vi "Main Loop.vi"(8 "error in (no error)":errorcluster, 10 "Chart Notifier":refnum<notifier>, 11 "Message Queues":T1) -> (0 "error out":errorcluster)   [LabVIEW 2018, in "4-20mA Module.lvlib" / "4-20mA Module Engine.lvlib"]
uses:
  4-20mA Module Engine.lvlib
  Pressure Regulator/Controls/4-20mA Message Queues.ctl
  support/Message Queue/Message Cluster.ctl
  State Cluster.ctl
  State Enum.ctl
  Pressure Transmitter/Pressure Transmitter Device Settings.ctl
  Pressure Reg Module/Pressure Regulator Device Settings.ctl
  Measure Instrument/PID 1 Parameters Cluster.ctl
  Pressure Regulator/Controls/4-20mA Display Cluster.ctl
  <vilib>/Platform/TimedLoop/XDataNode/timing_clust.ctl
  <vilib>/Platform/TimedLoop/XDataNode/nitl_modes.ctl
  <vilib>/Platform/TimedLoop/XDataNode/wakeup.ctl
  Tag VIs/Tag FGV Operation Enum.ctl
  Pressure Regulator/Controls/4-20mA Module Settings Cluster.ctl
  support/Message Queue/Enqueue Message (Single).vi
  <vilib>/Utility/error.llb/Error Cluster From Error Code.vi
  <vilib>/Platform/TimedLoop/XDataNode/XDataNode.xnode
  <vilib>/ErrorRing/Error Ring.xnode
  support/Message Queue/Message Queue.lvlib
  <vilib>/Platform/TimedLoop/XDataNode/XDNodeRunTimeDep.lvlib
  Shared Variables/Dynamic Shared Variables.lvlib
  Pressure Transmitter/Pressure Transmitter Library.lvlib
  Pressure Reg Module/Pressure Regulator Library.lvlib
  Pressure Regulator/4-20mA Module.lvlib
panel:
  out "Period (s)":dbl format="%_4g"
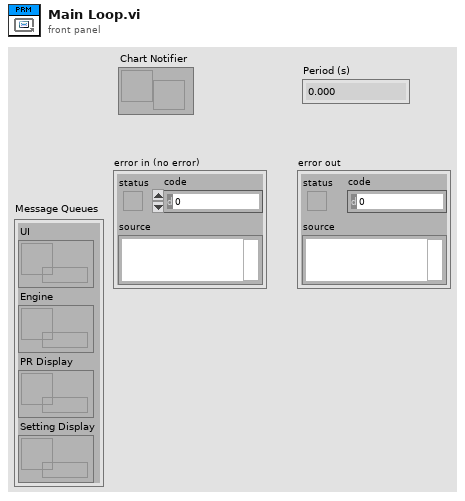
[diagram p1: front panel]
types:
  T1 = typedef "4-20mA Module.lvlib/4-20mA Message Queues.ctl" = cluster{"UI":refnum<queue>, "Engine":refnum<queue>, "PR Display":refnum<queue>, "Setting Display":refnum<queue>}
  T2 = typedef "4-20mA Module.lvlib/4-20mA Display Cluster.ctl" = cluster{"Input 4-20":dbl, "Output 4-20":dbl, "Cycle Period":dbl, "Status":enum16{"Off", "On", "Not Initialized"}}
  T3 = typedef "XDNodeRunTimeDep.lvlib/timing_clust.ctl" = cluster{"Expected End [f-1]":u64, "Actual End [f-1]":u64, "Finished Late? [f-1]":bool, "Expected End [i-1]":u64, "Actual End [i-1]":u64, "Finished Late? [i-1]":bool, "Expected Start [i]":u64, "Actual Start [i]":u64, "Expected Start [f]":u64, "Actual Start [f]":u64, "Source Name":string, "Structure Name":string, "Period":i64, "Deadline":i64, "Offset":i64, "Start":i64, "Priority":i32, "Timeout":i32, "Mode":T4, "Wakeup Reason":T5, "Error":errorcluster, "Source Type":string, "Secondary Source Type":string, "Global End Time":u64, "Global Start Time":u64, "Frame Duration":u64, "Iteration Duration":u64, "Assigned CPU":i32, "I/O Scan Engine Mode":u32}
  T4 = typedef "XDNodeRunTimeDep.lvlib/nitl_modes.ctl" = enum32{"No Change", "Process missed periods, maintain original phase", "Discard missed periods, maintain original phase", "Process missed periods, ignore original phase", "Discard missed periods, ignore original phase"}
  T5 = typedef "XDNodeRunTimeDep.lvlib/wakeup.ctl" = enum32{"Normal", "Aborted", "Asynchronous wakeup", "Timing source error", "Timed loop error", "Timeout"}
  T6 = cluster{"enable? (F)":bool, "name":string, "alarm on":bool, "priority":u32, "ack type":enum16{"Auto", "User", "None", "Each Occurrence"}, "area":string, "description":string, "log? (T)":bool}
  T7 = typedef "Tag FGV Operation Enum.ctl" = enum16{"Init", "Set Notification Queue", "Create Tag", "Commit", "Write Tag (Numeric)", "Write Tag (Boolean)", "Read All Tags", "Read One Tag", "Delete Tag Category", "Set Alarm Parameters (Numeric)", "Set Alarm Parameters (Boolean)", "Enable All Alarms", "Disable All Alarms", "Delete All Tags", "Read Alarms", "Ack Alarm"}
  T8 = enum32{"u32BitField", "bool", "double", "string", "int8", "uint8", "int16", "uint16", "int32", "uint32", "int64", "uint64", "single", "double waveform", "int16 waveform", "array of boolean", "array of int8", "array of uint8", "array of int16", "array of uint16", "array of int32", "array of uint32", "array of int64", "array of uint64", "array of single", "array of double", "array of double waveform", "array of int16 waveform", "array of string", "variant", "timestamp", "fixed point", "custom"}
  T9 = typedef "4-20mA Module.lvlib/4-20mA Module Engine.lvlib/State Enum.ctl" = enum16{"Measuring", "Idle", "Paused"}
  T10 = typedef "4-20mA Module.lvlib/4-20mA Module Settings Cluster.ctl" = cluster{"Cycle Period":dbl, "PID 2 Parameters":cluster{"Input Device":enum16{"Default", "4-20mA"}, "Output Device":enum16{"Default", "Equilibar Pressure Reg", "Flow Regulator"}, "Setpoint":dbl, "PID gains":cluster{"proportional gain (Kc)":dbl, "integral time (Ti, min)":dbl, "derivative time (Td, min)":dbl}, "output range":cluster{"output low":dbl, "output high":dbl}}, "Manual Entry":dbl, "Auto?":bool, "4-20mA Input Settings":T11, "4-20mA Out Settings":T12, "Input Channel Tag Name ":string}
  T11 = typedef "Pressure Transmitter Library.lvlib/Pressure Transmitter Device Settings.ctl" = cluster{"Input Channel ":u16}
  T12 = typedef "Pressure Regulator Library.lvlib/Pressure Regulator Device Settings.ctl" = cluster{"Output DAQ Task":refnum<k21>}
  T13 = typedef "4-20mA Module.lvlib/4-20mA Module Engine.lvlib/State Cluster.ctl" = cluster{"State":T9, "Start Time":timestamp, "Configuration":cluster{"Cycle Period":dbl, "PID 2 Parameters":cluster{"Input Device":enum16{"Default", "4-20mA"}, "Output Device":enum16{"Default", "Equilibar Pressure Reg", "Flow Regulator"}, "Setpoint":dbl, "PID gains":cluster{"proportional gain (Kc)":dbl, "integral time (Ti, min)":dbl, "derivative time (Td, min)":dbl}, "output range":cluster{"output low":dbl, "output high":dbl}}, "Manual Entry":dbl, "Auto?":bool, "4-20mA Input Settings":T11, "4-20mA Out Settings":T12, "Input Channel Tag Name ":string}, "Current Time":timestamp, "PID 1 Parameters":T14, "First Iteration":bool, "Data":cluster{"4-20mA Input":dbl, "PID 2 Process Variable":dbl, "PID 2 Output":dbl, "4-20mA Output":dbl}, "Process Name":string, "Pump On?":enum16{"Off", "On", "Not Initialized"}, "Input Error":bool, "Output Error":bool, "Log Started":bool, "Current Setpoint":dbl}
  T14 = typedef "PID 1 Parameters Cluster.ctl" = cluster{"Setpoint":dbl, "PID gains":cluster{"proportional gain (Kc)":dbl, "integral time (Ti, min)":dbl, "derivative time (Td, min)":dbl}}
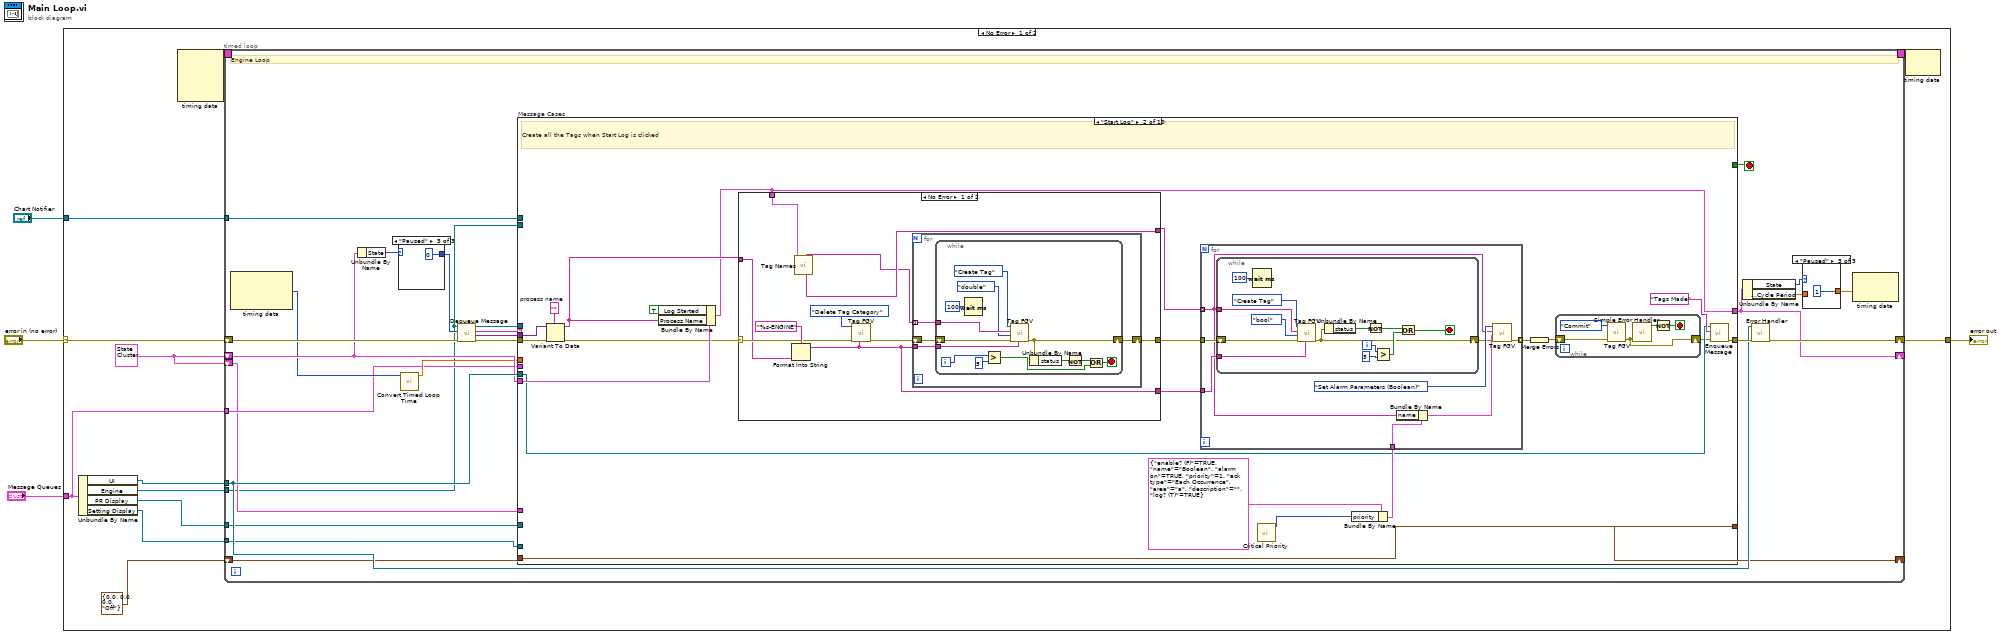
[diagram p0: block diagram]
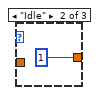
[diagram p3: hidden frame]
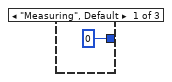
[diagram p4: hidden frame]
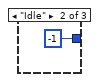
[diagram p5: hidden frame]
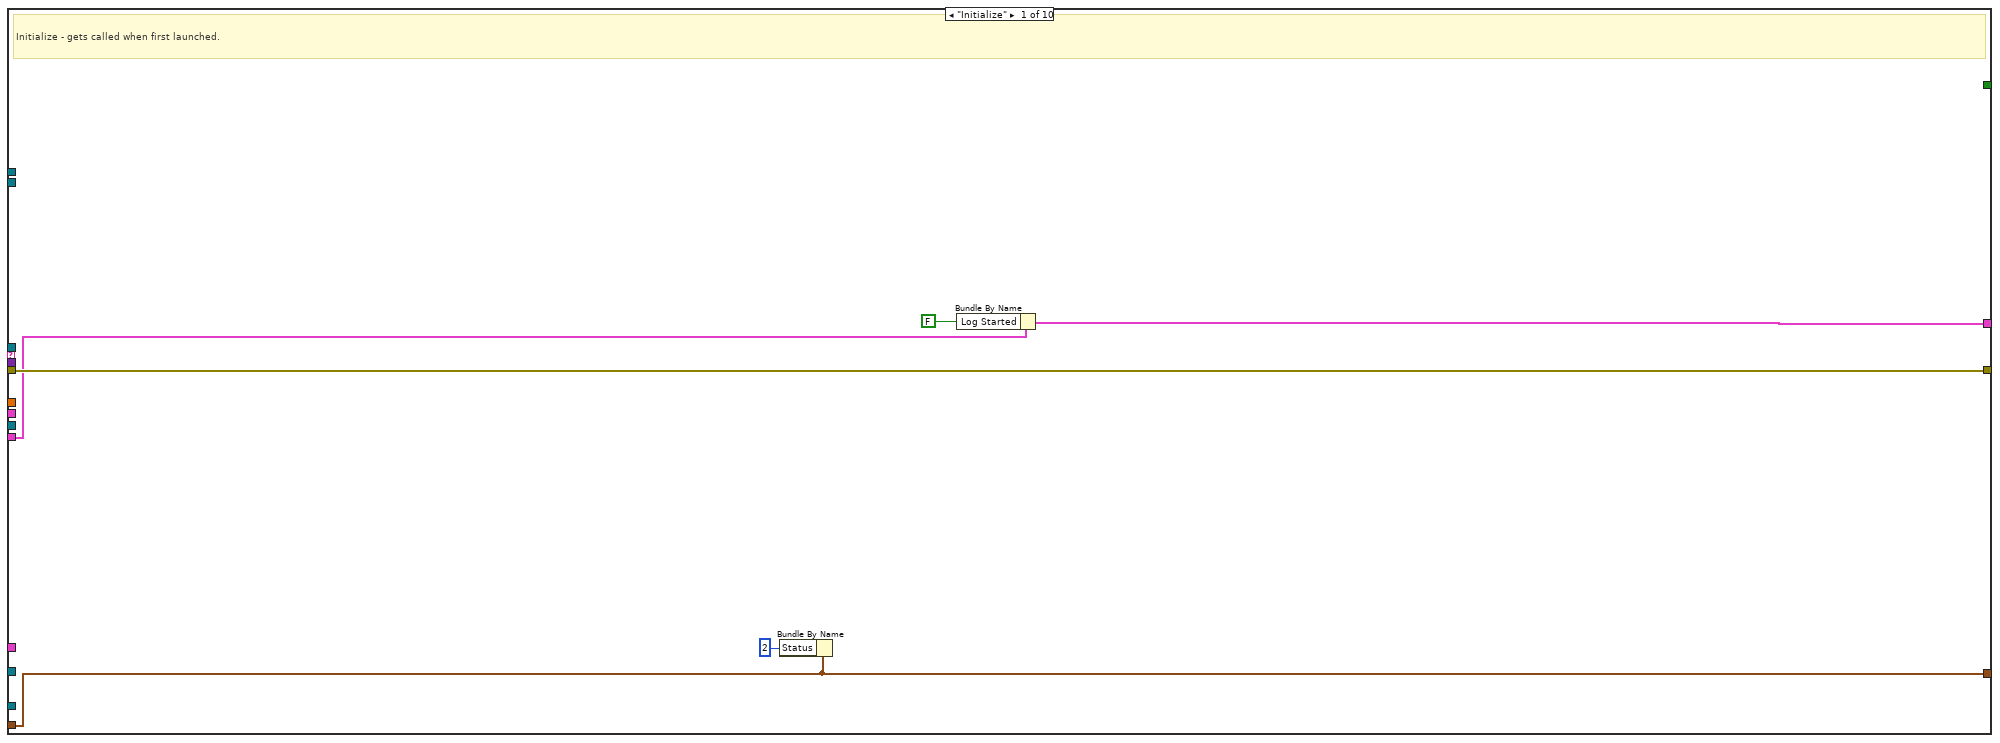
[diagram p6: hidden frame]
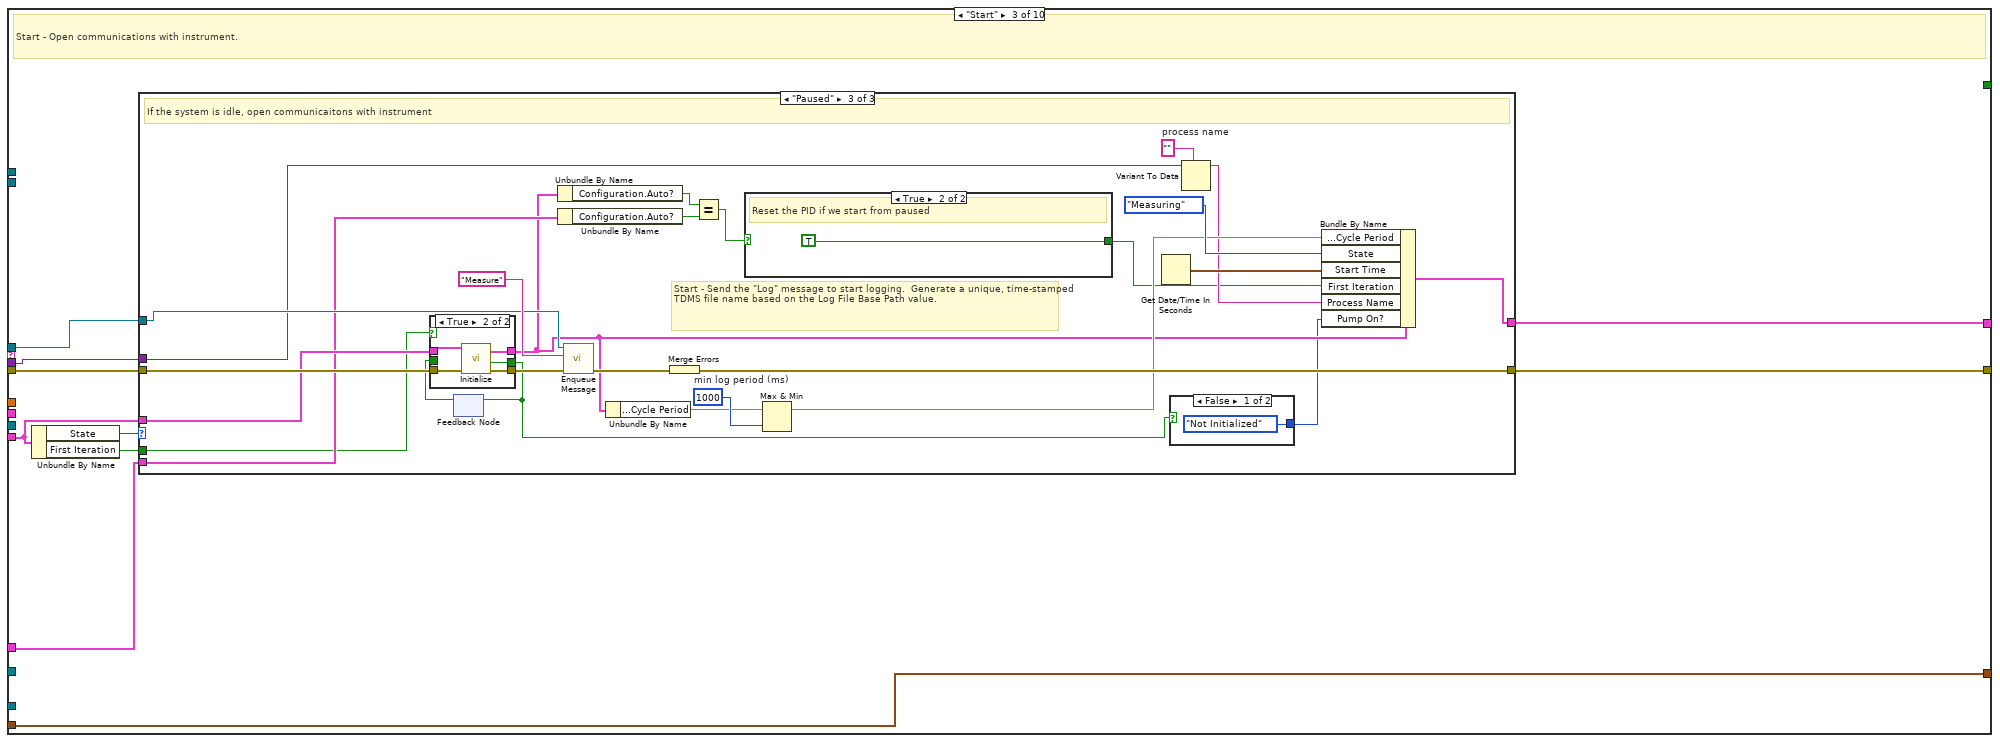
[diagram p8: hidden frame]
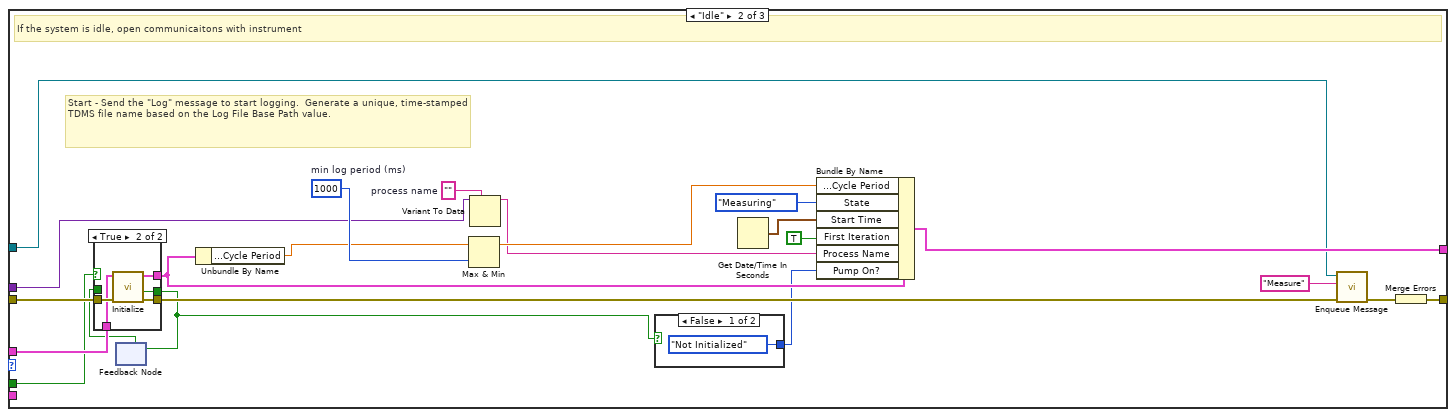
[diagram p10: hidden frame]
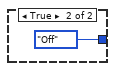
[diagram p12: hidden frame]
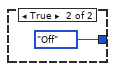
[diagram p14: hidden frame]
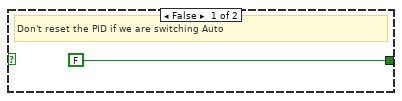
[diagram p15: hidden frame]
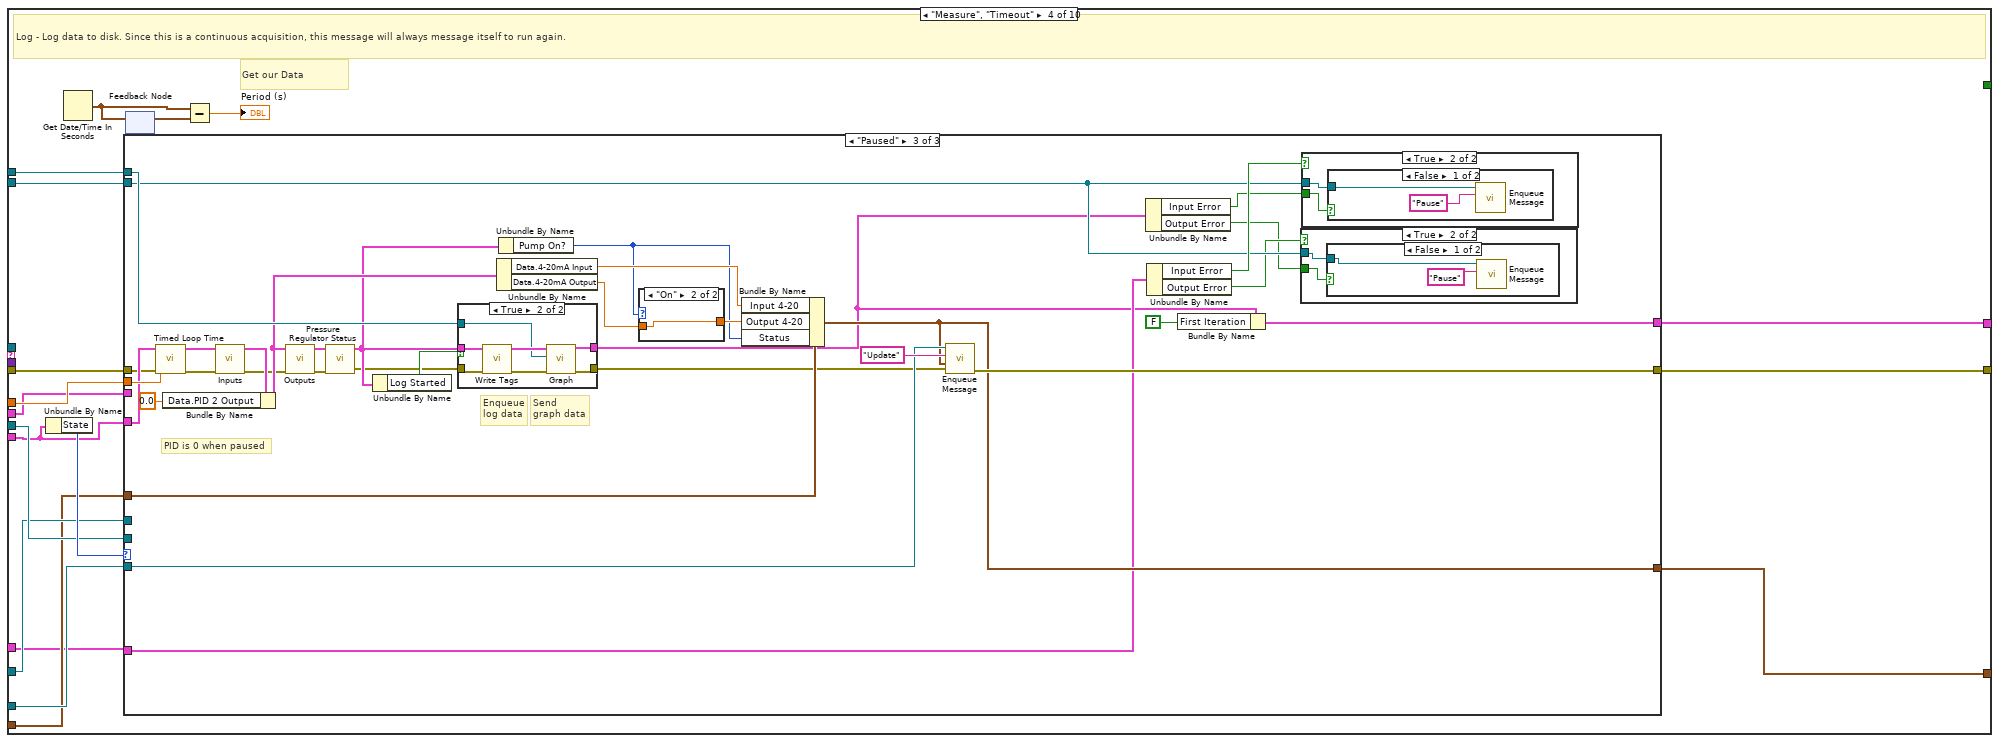
[diagram p16: hidden frame]
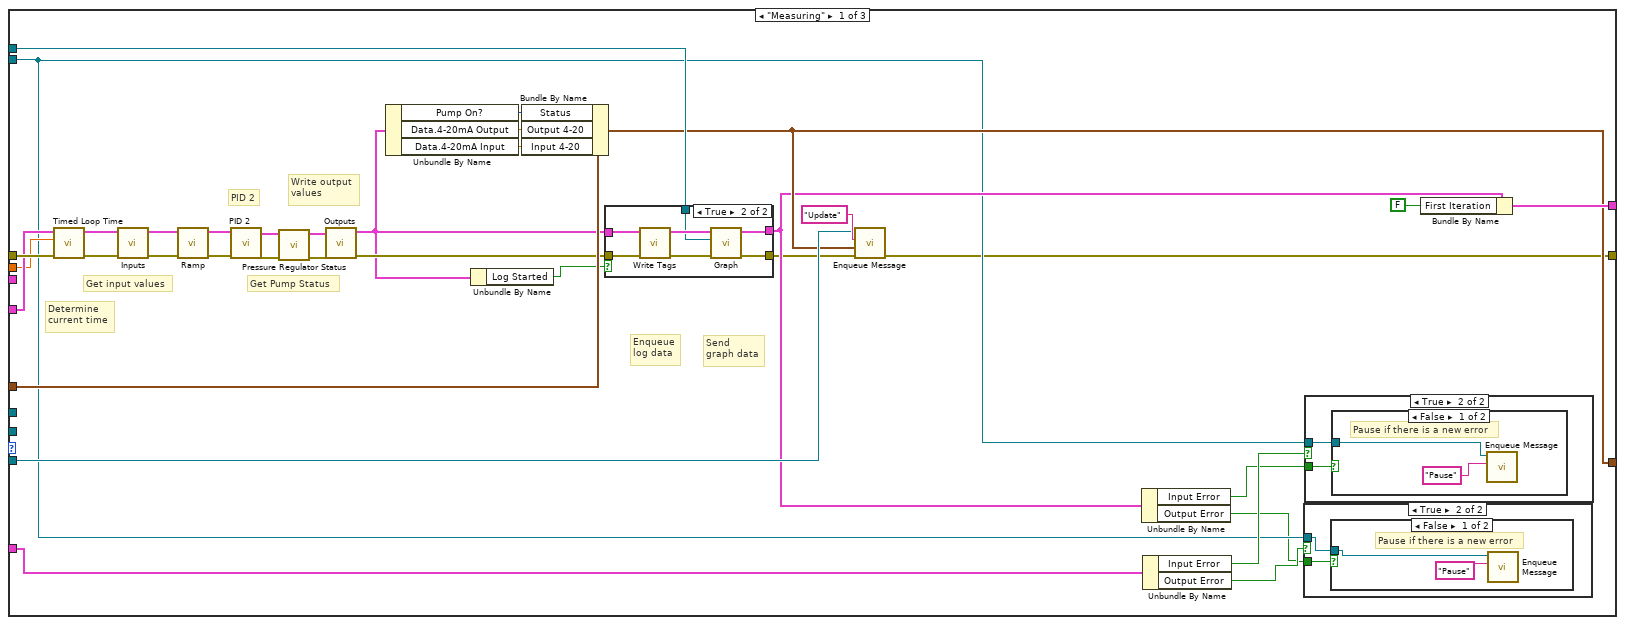
[diagram p17: hidden frame]
diagram:
  n1 = case shown="No Error" "error in (no error)" {
    selector: "error in (no error)" -> [w15 w454]
    tunnel: "Message Queues" -> [w11 _]
    tunnel: [w16 w454] -> w3
    tunnel: "Chart Notifier" -> [w9 _]
    frame No Error {
      w6 = T13 {"State"=enum."Idle", "Start Time"=timestamp(0 s since 1904-01-01), "Configuration"={"Cycle Period"=0.0, "PID 2 Parameters"={"Input Device"=enum."4-20mA", "Output Device"=enum."Equilibar Pressure Reg", "Setpoint"=0.0, "PID gains"={"proportional gain (Kc)"=1.0, "integral time (Ti, min)"=0.01, "derivative time (Td, min)"=0.0}, "output range"={"output low"=0.0, "output high"=100.0}}, "Manual Entry"=0.0, "Auto?"=TRUE, "4-20mA Input Settings"={"Input Channel "=0}, "4-20mA Out Settings"={"Output DAQ Task"=""}, "Input Channel Tag Name "=""}, "Current Time"=timestamp(0 s since 1904-01-01), "PID 1 Parameters"={"Setpoint"=0.0, "PID gains"={"proportional gain (Kc)"=1.0, "integral time (Ti, min)"=0.01, "derivative time (Td, min)"=0.0}}, "First Iteration"=FALSE, "Data"={"4-20mA Input"=0.0, "PID 2 Process Variable"=0.0, "PID 2 Output"=0.0, "4-20mA Output"=0.0}, "Process Name"="", "Pump On?"=enum."Off", "Input Error"=FALSE, "Output Error"=FALSE, "Log Started"=FALSE, "Current Setpoint"=0.0} ("State")
      n2 = Unbundle By Name(w11) -> ("UI"=w14:refnum<queue>, "Engine"=w10:refnum<queue>, "PR Display"=w8:refnum<queue>, "Setting Display"=w7:refnum<queue>)
      n3 = node-c288() -> (w13:T3)  [unwired: 4 in]
      n4 = timed-loop {
        tunnel: w10 -> [w19]
        shift-right: [w17] -> _
        shift-left: w6 -> [w34]
        shift-right: [w36] -> w16
        shift-left: w15 -> [w42]
        tunnel: w14 -> [w35]
        timing: w13 -> [_]
        timing-out: [_] -> w12
        tunnel: w11 -> [w26]
        tunnel: w9 -> [w25]
        tunnel: w8 -> [w24]
        tunnel: w7 -> [w23]
        shift-right: [w22] -> _
        shift-left: T2 {"Input 4-20"=0.0, "Output 4-20"=0.0, "Cycle Period"=0.0, "Status"=enum."Off"} ("PRM Display Cluster") -> [w18]
        shift-left: w6 -> [w21]
        stop <- w20 stop-if-true
        # "Engine Loop"
        n5 = node-c288() -> (w28:i64)  [unwired: 1 in, 2 out]
        n6 = Unbundle By Name(w34) -> ("State"=w33:T9)
        n7 = case shown="\"Paused\"" w33 {
          tunnel: [0 ("timeout in ms (-1)") -1 ("timeout in ms (-1)") 0 ("timeout in ms (-1)")] -> w32
          frame "Measuring", Default {
          }
          frame "Idle" {
          }
          frame "Paused" {
          }
        }
        n8 = call "Convert Timed Loop Time.vi"("Actual Start [i]"=w28) -> ("ET since start (s)"=w27:dbl)  [unwired: 10 in]
        n9 = call "Dequeue Message.vi"("error in (no error)"=w42, "timeout in ms (-1)"=w32, "Message Queue"=w19) -> ("error out"=w41:errorcluster, "Message Data"=w39:variant, "Message"=w40:string, "dup Message Queue"=w38:refnum<queue>)  [unwired: 5 in]
        n10 = case "Message Cases" shown="\"Start Log\"" w40 {
          selector: w40 -> [_ _ _ _ _ _ _ _ _ w443]
          tunnel: w38 -> [_ _ w143 _ w362 _ _ w430 _ _]
          tunnel: w41 -> [w59 w77 w142 w231 w351 w377 w424 w433 w440 _]
          tunnel: [w59 w63 w144 w232 w355 w381 w422 w435 w439 w444] -> w37
          tunnel: w34 -> [w58 w76 w139 w230 w350 w379 w421 w426 w437 w441]
          tunnel: [_ _ _ _ _ _ _ TRUE _ _] -> w20
          tunnel: w39 -> [_ w78 w140 _ _ _ w425 _ _ _]
          tunnel: w35 -> [_ w64 _ w233 w361 w386 _ w434 _ _]
          tunnel: w27 -> [_ _ _ w229 _ _ _ _ _ _]
          tunnel: w26 -> [_ _ _ w228 _ _ _ _ _ _]
          tunnel: w25 -> [_ _ _ w224 _ _ _ _ _ _]
          tunnel: w24 -> [_ _ _ w223 w353 _ _ _ _ _]
          tunnel: w23 -> [_ _ _ w222 w354 w383 _ _ _ _]
          tunnel: w18 -> [w55 w80 w138 w221 w352 w380 w423 w427 w438 w442]
          tunnel: [w55 w80 w138 w220 w352 w380 w423 w427 w438 w442] -> w22
          tunnel: w21 -> [_ _ w137 w219 _ _ _ _ _ _]
          tunnel: w19 -> [_ _ _ w218 _ _ _ _ _ _]
          tunnel: [w56 w62 w135 w217 w349 w374 w418 w426 w437 w441] -> w17
          frame "Initialize" {
            # "Initialize - gets called when first launched."
            n11 = Bundle By Name(cluster=w55, "Status"=u16 2) -> ()  [unwired: 1 out]
            n12 = Bundle By Name(cluster=w58, "Log Started"=FALSE) -> (w56:T13)
          }
          frame "Start Log" {
            w79 = ""  # process name
            # "Create all the Tags when Start Log is clicked"
            n13 = Variant To Data(error in=w77, type=w79, Variant=w78) -> (data=w74:string, error out=w75:errorcluster)
            n14 = Bundle By Name(cluster=w76, "Log Started"=TRUE, "Process Name"=w74) -> (w62:T13)
            n15 = case shown="No Error" w75 {
              selector: w75 -> [w113 w134]
              tunnel: [w116 w134] -> w69
              tunnel: w74 -> [w111 _]
              tunnel: [w110 _] -> w70
              tunnel: [w109 _] -> w67
              tunnel: w62 -> [w108 _]
              frame No Error {
                n16 = Format Into String(format string="%s-ENGINE", w111) -> (resulting string=w109:string)  [unwired: 2 in, 1 out]
                n17 = call "Tag Names.vi"("State in"=w108) -> ("All Boolean Tags"=w110:string[], "All  Numeric Tags"=w107:string[])  [unwired: 8 in, 1 out]
                n18 = call "Tag FGV.vi"("Tag Category"=w109, "error in (no error)"=w113, "Operation"=Tag_FGV_Operation_Enum."Delete Tag Category") -> ("error out"=w112:errorcluster)  [unwired: 3 in, 5 out]
                n19 = for {
                  tunnel: w107 -> [w120] mode=indexing
                  shift-right: [w118] -> w116
                  shift-left: w112 -> [w119]
                  tunnel: w109 -> [w117]
                  n20 = while {
                    tunnel: w120 -> [w132]
                    tunnel: w117 -> [w129]
                    shift-right: [w128] -> w118
                    shift-left: w119 -> [w130]
                    i -> [w123]
                    stop <- w121 stop-if-true
                    n21 = Wait (ms)(milliseconds to wait=u32 100) -> ()  [unwired: 1 out]
                    n22 = Greater?(x=w123, y=5 ("x")) -> (0:w122:bool)
                    n23 = call "Tag FGV.vi"("Tag Category"=w129, "error in (no error)"=w130, "Data"=T8."double" ("data type"), "Tag Name"=w132, "Operation"=Tag_FGV_Operation_Enum."Create Tag") -> ("error out"=w128:errorcluster)  [unwired: 1 in, 5 out]
                    n24 = Unbundle By Name(w128) -> ("status"=w127:bool)
                    n25 = Not(x=w127) -> (.not. x?=w125:bool)
                    n26 = Or(x=w125, y=w122) -> (x .or. y?=w121:bool)
                  }
                }
              }
              frame Error {
              }
            }
            n27 = call "Critical Priority.vi"() -> ("critical priority"=w72:i32)  [unwired: 11 in]
            n28 = Bundle By Name(cluster=T6 {"enable? (F)"=TRUE, "name"="Boolean", "alarm on"=TRUE, "priority"=1, "ack type"=enum."Each Occurrence", "area"="a", "description"="", "log? (T)"=TRUE} ("Boolean alarm settings"), "priority"=w72) -> (w71:T6)
            n29 = for {
              tunnel: w71 -> [w93]
              tunnel: [w92] -> w68 mode=indexing
              tunnel: w70 -> [w86] mode=indexing
              tunnel: w69 -> [w88]
              tunnel: w67 -> [w89]
              n30 = while {
                tunnel: w86 -> [w105]
                tunnel: w89 -> [w102]
                shift-right: [w94] -> w87
                shift-left: w88 -> [w103]
                i -> [w97]
                stop <- w95 stop-if-true
                n31 = Wait (ms)(milliseconds to wait=u32 100) -> ()  [unwired: 1 out]
                n32 = call "Tag FGV.vi"("Tag Category"=w102, "error in (no error)"=w103, "Data"=T8."bool" ("data type"), "Tag Name"=w105, "Operation"=Tag_FGV_Operation_Enum."Create Tag") -> ("error out"=w94:errorcluster)  [unwired: 1 in, 5 out]
                n33 = Unbundle By Name(w94) -> ("status"=w101:bool)
                n34 = Not(x=w101) -> (.not. x?=w99:bool)
                n35 = Greater?(x=w97, y=5 ("x")) -> (0:w96:bool)
                n36 = Or(x=w99, y=w96) -> (x .or. y?=w95:bool)
              }
              n37 = Bundle By Name(cluster=w93, "name"=w86) -> (w91:T6)
              n38 = call "Tag FGV.vi"("error in (no error)"=w87, "Data"=w91, "Tag Name"=w86, "Operation"=Tag_FGV_Operation_Enum."Set Alarm Parameters (Boolean)") -> ("error out"=w92:errorcluster)  [unwired: 2 in, 5 out]
            }
            n39 = Merge Errors(w68) -> (w61:errorcluster)
            n40 = while {
              shift-right: [w83] -> w60
              shift-left: w61 -> [w84]
              stop <- w81 stop-if-true
              n41 = call "Tag FGV.vi"("error in (no error)"=w84, "Operation"=Tag_FGV_Operation_Enum."Commit") -> ("error out"=w83:errorcluster)  [unwired: 4 in, 5 out]
              n42 = call <vilib>:"Simple Error Handler.vi"("error in (no error)"=w83) -> ("error?"=w82:bool)  [unwired: 4 in, 4 out]
              n43 = Not(x=w82) -> (.not. x?=w81:bool)
            }
            n44 = call-poly "Enqueue Message.vi"("error in (no error)"=w60, "Message"="Tags Made", "Message Queue"=w64) -> ("error out"=w63:errorcluster)  [unwired: 7 in, 1 out]
          }
          frame "Start" {
            # "Start - Open communications with instrument."
            n45 = Unbundle By Name(w139) -> ("State"=w141:T9, "First Iteration"=w136:bool)
            n46 = case shown="\"Paused\"" w141 {
              tunnel: [w145 w168 w204] -> w144
              tunnel: w143 -> [_ w159 w195]
              tunnel: w142 -> [w145 w157 w193]
              tunnel: w139 -> [w146 w156 w192]
              tunnel: [w146 w166 w202] -> w135
              tunnel: w140 -> [_ w154 w190]
              tunnel: w137 -> [_ _ w186]
              tunnel: w136 -> [_ w147 w181]
              frame "Measuring", Default {
                # "The system is already running. Ignore the \"Start\" message."
              }
              frame "Idle" {
                w155 = ""  # process name
                w163 = 1000  # min log period (ms)
                # "Start - Send the \"Log\" message to start logging.  Generate a unique, time-stamped TDMS file name based on the Log File Base Path value."
                # "If the system is idle, open communicaitons with instrument"
                n47 = feedback #1() -> (w149:bool)  [unwired: 1 in]
                n48 = case shown="True" w147 {
                  tunnel: w157 -> [w170 w176]
                  tunnel: w156 -> [w171 w175]
                  tunnel: [w171 w174] -> w152
                  tunnel: [w170 w173] -> w151
                  tunnel: [w169 w172] -> w148
                  tunnel: w149 -> [w169 _]
                  frame False {
                  }
                  frame True {
                    n49 = call "Initialize.vi"("error in (no error)"=w176, "State in"=w175) -> ("error out"=w173:errorcluster, "Pump Initialized"=w172:bool, "State out"=w174:T13)  [unwired: 7 in]
                  }
                }
                n50 = feedback-in #1(w148) -> ()
                n51 = Unbundle By Name(w152) -> ("Configuration.Cycle Period"=w162:dbl)
                n52 = Max & Min(x=w162, y=w163) -> (max(x,y)=w161:dbl)  [unwired: 1 out]
                n53 = Variant To Data(type=w155, Variant=w154) -> (data=w153:string)  [unwired: 1 in, 1 out]
                n54 = case shown="False" w148 {
                  tunnel: [enum16{"Off", "On", "Not Initialized"}."Not Initialized" ("Pump On?") enum16{"Off", "On", "Not Initialized"}."Off" ("Pump On?")] -> w150
                  frame False {
                  }
                  frame True {
                  }
                }
                n55 = Get Date/Time In Seconds() -> (seconds since 1Jan1904=w160:timestamp)
                n56 = Bundle By Name(cluster=w152, "Configuration.Cycle Period"=w161, "State"=State_Enum."Measuring", "Start Time"=w160, "First Iteration"=TRUE, "Process Name"=w153, "Pump On?"=w150) -> (w166:T13)
                n57 = call-poly "Enqueue Message.vi"("error in (no error)"=w151, "Message"="Measure", "Message Queue"=w159) -> ("error out"=w164:errorcluster)  [unwired: 7 in, 1 out]
                n58 = Merge Errors(w164) -> (w168:errorcluster)
              }
              frame "Paused" {
                w191 = ""  # process name
                w199 = 1000  # min log period (ms)
                # "Start - Send the \"Log\" message to start logging.  Generate a unique, time-stamped TDMS file name based on the Log File Base Path value."
                # "If the system is idle, open communicaitons with instrument"
                n59 = feedback #2() -> (w180:bool)  [unwired: 1 in]
                n60 = case shown="True" w181 {
                  tunnel: [w207 w212] -> w194
                  tunnel: w193 -> [w207 w211]
                  tunnel: w192 -> [w206 w210]
                  tunnel: [w206 w209] -> w183
                  tunnel: [w205 w208] -> w179
                  tunnel: w180 -> [w205 _]
                  frame False {
                  }
                  frame True {
                    n61 = call "Initialize.vi"("error in (no error)"=w211, "State in"=w210) -> ("error out"=w212:errorcluster, "Pump Initialized"=w208:bool, "State out"=w209:T13)  [unwired: 7 in]
                  }
                }
                n62 = feedback-in #2(w179) -> ()
                n63 = Unbundle By Name(w183) -> ("Configuration.Auto?"=w187:bool)
                n64 = Unbundle By Name(w186) -> ("Configuration.Auto?"=w185:bool)
                n65 = call-poly "Enqueue Message.vi"("error in (no error)"=w194, "Message"="Measure", "Message Queue"=w195) -> ("error out"=w200:errorcluster)  [unwired: 7 in, 1 out]
                n66 = Unbundle By Name(w183) -> ("Configuration.Cycle Period"=w198:dbl)
                n67 = Merge Errors(w200) -> (w204:errorcluster)
                n68 = Equal?(x=w187, y=w185) -> (x = y?=w188:bool)
                n69 = case shown="True" w188 {
                  tunnel: [FALSE ("First Iteration") TRUE ("First Iteration")] -> w184
                  frame False {
                    # "Don't reset the PID if we are switching Auto"
                  }
                  frame True {
                    # "Reset the PID if we start from paused"
                  }
                }
                n70 = Max & Min(x=w198, y=w199) -> (max(x,y)=w197:dbl)  [unwired: 1 out]
                n71 = Get Date/Time In Seconds() -> (seconds since 1Jan1904=w196:timestamp)
                n72 = case shown="False" w179 {
                  tunnel: [enum16{"Off", "On", "Not Initialized"}."Not Initialized" ("Pump On?") enum16{"Off", "On", "Not Initialized"}."Off" ("Pump On?")] -> w182
                  frame False {
                  }
                  frame True {
                  }
                }
                n73 = Variant To Data(type=w191, Variant=w190) -> (data=w189:string)  [unwired: 1 in, 1 out]
                n74 = Bundle By Name(cluster=w183, "Configuration.Cycle Period"=w197, "State"=State_Enum."Measuring", "Start Time"=w196, "First Iteration"=w184, "Process Name"=w189, "Pump On?"=w182) -> (w202:T13)
              }
            }
          }
          frame "Measure", "Timeout" {
            # "Get our Data"
            # "Log - Log data to disk. Since this is a continuous acquisition, this message will always message itself to run again."
            n75 = Unbundle By Name(w230) -> ("State"=w234:T9)
            n76 = Get Date/Time In Seconds() -> (seconds since 1Jan1904=w226:timestamp)
            n77 = case shown="\"Paused\"" w234 {
              tunnel: w231 -> [w269 w288 w311]
              tunnel: w230 -> [w268 w291 w312]
              tunnel: w233 -> [_ _ _]
              tunnel: [w249 w287 w323] -> w232
              tunnel: [w266 w291 w310] -> w217
              tunnel: w229 -> [w267 _ w328]
              tunnel: w228 -> [_ _ _]
              tunnel: w224 -> [w264 _ w329]
              tunnel: w223 -> [_ w292 _]
              tunnel: w222 -> [w262 w293 w325]
              tunnel: w221 -> [w261 w290 w326]
              tunnel: [w260 w290 w322] -> w220
              tunnel: w219 -> [w241 _ w319]
              tunnel: w218 -> [w256 _ w316]
              frame "Measuring" {
                # "Get Pump Status"
                # "Send\ngraph data"
                # "Enqueue\nlog data"
                # "PID 2"
                # "Determine\ncurrent time"
                # "Write output\nvalues"
                # "Get input values"
                n78 = call "Timed Loop Time.vi"("error in (no error)"=w269, "ET since start (s)"=w267, "State in"=w268) -> ("error out"=w242:errorcluster, "State out"=w243:T13)  [unwired: 7 in]
                n79 = call "Inputs.vi"("error in (no error)"=w242, "State in"=w243) -> ("error out"=w238:errorcluster, "State out"=w240:T13)  [unwired: 8 in]
                n80 = call "Ramp.vi"("error in (no error)"=w238, "New State"=w240) -> ("error out"=w237:errorcluster, "State"=w239:T13)  [unwired: 8 in]
                n81 = call "PID 2.vi"("error in (no error)"=w237, "State in"=w239) -> ("error out"=w247:errorcluster, "State out"=w248:T13)  [unwired: 8 in]
                n82 = call "Pressure Regulator Status.vi"("error in (no error)"=w247, "State In"=w248) -> ("error out"=w246:errorcluster, "State Out"=w245:T13)  [unwired: 8 in]
                n83 = call "Outputs.vi"("error in (no error)"=w246, "State in"=w245) -> ("error out"=w251:errorcluster, "State out"=w244:T13)  [unwired: 8 in]
                n84 = Unbundle By Name(w244) -> ("Pump On?"=w236:enum16{"Off", "On", "Not Initialized"}, "Data.4-20mA Output"=w252:dbl, "Data.4-20mA Input"=w235:dbl)
                n85 = Unbundle By Name(w244) -> ("Log Started"=w253:bool)
                n86 = Bundle By Name(cluster=w261, "Status"=w236, "Output 4-20"=w252, "Input 4-20"=w235) -> (w260:T2)
                n87 = case shown="True" w253 {
                  tunnel: [w271 w276] -> w250
                  tunnel: w264 -> [_ w275]
                  tunnel: w244 -> [w270 w274]
                  tunnel: w251 -> [w271 w273]
                  tunnel: [w270 w272] -> w257
                  frame False {
                  }
                  frame True {
                    n88 = call "Write Tags.vi"("error in (no error)"=w273, "State in"=w274) -> ("error out"=w277:errorcluster, "State out"=w278:T13)  [unwired: 8 in]
                    n89 = call "Graph.vi"("error in (no error)"=w277, "notifier out"=w275, "State in"=w278) -> ("error out"=w276:errorcluster, "State out"=w272:T13)  [unwired: 7 in]
                  }
                }
                n90 = call-poly "Enqueue Message.vi"("error in (no error)"=w250, "Message Data"=w260, "Message"="Update", "Message Queue"=w262) -> ("error out"=w249:errorcluster)  [unwired: 6 in, 1 out]
                n91 = Unbundle By Name(w257) -> ("Input Error"=w258:bool, "Output Error"=w254:bool)
                n92 = Unbundle By Name(w241) -> ("Input Error"=w259:bool, "Output Error"=w255:bool)
                n93 = case shown="True" w255 {
                  tunnel: w254 -> [_ w280]
                  tunnel: w256 -> [_ w279]
                  frame False {
                  }
                  frame True {
                    n94 = case shown="False" w280 {
                      tunnel: w279 -> [w282 _]
                      frame False {
                        # "Pause if there is a new error"
                        n95 = call-poly "Enqueue Message.vi"("Message"="Pause", "Message Queue"=w282) -> ()  [unwired: 8 in, 2 out]
                      }
                      frame True {
                      }
                    }
                  }
                }
                n96 = case shown="True" w259 {
                  tunnel: w258 -> [_ w284]
                  tunnel: w256 -> [_ w283]
                  frame False {
                  }
                  frame True {
                    n97 = case shown="False" w284 {
                      tunnel: w283 -> [w286 _]
                      frame False {
                        # "Pause if there is a new error"
                        n98 = call-poly "Enqueue Message.vi"("Message"="Pause", "Message Queue"=w286) -> ()  [unwired: 8 in, 2 out]
                      }
                      frame True {
                      }
                    }
                  }
                }
                n99 = Bundle By Name(cluster=w257, "First Iteration"=FALSE) -> (w266:T13)
              }
              frame "Idle", Default {
                n100 = call-poly "Enqueue Message.vi"("error in (no error)"=w288, "Message"="Update", "Message Queue"=w292) -> ("error out"=w289:errorcluster)  [unwired: 7 in, 1 out]
                n101 = call-poly "Enqueue Message.vi"("error in (no error)"=w289, "Message Data"=w290, "Message"="Update", "Message Queue"=w293) -> ("error out"=w287:errorcluster)  [unwired: 6 in, 1 out]
              }
              frame "Paused" {
                # "PID is 0 when paused"
                # "Send\ngraph data"
                # "Enqueue\nlog data"
                n102 = call "Timed Loop Time.vi"("error in (no error)"=w311, "ET since start (s)"=w328, "State in"=w312) -> ("error out"=w299:errorcluster, "State out"=w301:T13)  [unwired: 7 in]
                n103 = call "Inputs.vi"("error in (no error)"=w299, "State in"=w301) -> ("error out"=w298:errorcluster, "State out"=w300:T13)  [unwired: 8 in]
                n104 = Bundle By Name(cluster=w300, "Data.PID 2 Output"=0.0 ("Data.PID 2 output")) -> (w308:T13)
                n105 = call "Outputs.vi"("error in (no error)"=w298, "State in"=w308) -> ("error out"=w304:errorcluster, "State out"=w297:T13)  [unwired: 8 in]
                n106 = call "Pressure Regulator Status.vi"("error in (no error)"=w304, "State In"=w297) -> ("error out"=w302:errorcluster, "State Out"=w303:T13)  [unwired: 8 in]
                n107 = Unbundle By Name(w303) -> ("Log Started"=w307:bool)
                n108 = case shown="True" w307 {
                  tunnel: w329 -> [_ w336]
                  tunnel: [w330 w335] -> w324
                  tunnel: w303 -> [w331 w334]
                  tunnel: w302 -> [w330 w333]
                  tunnel: [w331 w332] -> w305
                  frame False {
                  }
                  frame True {
                    n109 = call "Write Tags.vi"("error in (no error)"=w333, "State in"=w334) -> ("error out"=w338:errorcluster, "State out"=w337:T13)  [unwired: 8 in]
                    n110 = call "Graph.vi"("error in (no error)"=w338, "notifier out"=w336, "State in"=w337) -> ("error out"=w335:errorcluster, "State out"=w332:T13)  [unwired: 7 in]
                  }
                }
                n111 = Unbundle By Name(w308) -> ("Data.4-20mA Input"=w306:dbl, "Data.4-20mA Output"=w321:dbl)
                n112 = Unbundle By Name(w303) -> ("Pump On?"=w296:enum16{"Off", "On", "Not Initialized"})
                n113 = case shown="\"On\"" w296 {
                  tunnel: w321 -> [_ w348]
                  tunnel: [0.0 w348] -> w320
                  frame "Off", Default {
                  }
                  frame "On" {
                  }
                }
                n114 = Bundle By Name(cluster=w326, "Input 4-20"=w306, "Output 4-20"=w320, "Status"=w296) -> (w322:T2)
                n115 = call-poly "Enqueue Message.vi"("error in (no error)"=w324, "Message Data"=w322, "Message"="Update", "Message Queue"=w325) -> ("error out"=w323:errorcluster)  [unwired: 6 in, 1 out]
                n116 = Unbundle By Name(w305) -> ("Input Error"=w317:bool, "Output Error"=w314:bool)
                n117 = Unbundle By Name(w319) -> ("Input Error"=w318:bool, "Output Error"=w315:bool)
                n118 = Bundle By Name(cluster=w305, "First Iteration"=FALSE) -> (w310:T13)
                n119 = case shown="True" w315 {
                  tunnel: w314 -> [_ w340]
                  tunnel: w316 -> [_ w339]
                  frame False {
                  }
                  frame True {
                    n120 = case shown="False" w340 {
                      tunnel: w339 -> [w342 _]
                      frame False {
                        n121 = call-poly "Enqueue Message.vi"("Message"="Pause", "Message Queue"=w342) -> ()  [unwired: 8 in, 2 out]
                      }
                      frame True {
                      }
                    }
                  }
                }
                n122 = case shown="True" w318 {
                  tunnel: w317 -> [_ w344]
                  tunnel: w316 -> [_ w343]
                  frame False {
                  }
                  frame True {
                    n123 = case shown="False" w344 {
                      tunnel: w343 -> [w346 _]
                      frame False {
                        n124 = call-poly "Enqueue Message.vi"("Message"="Pause", "Message Queue"=w346) -> ()  [unwired: 8 in, 2 out]
                      }
                      frame True {
                      }
                    }
                  }
                }
              }
            }
            n125 = feedback-in #3(w226) -> ()
            n126 = feedback #3() -> (w227:timestamp)  [unwired: 1 in]
            n127 = Subtract(x=w226, y=w227) -> (x-y=→"Period (s)":dbl)
          }
          frame "Stop" {
            # "Stop - Flush the message queue of any pending \"Log\" messages. Call 'Flush Data to Log File.vi' so any pending data is not lost."
            n128 = Unbundle By Name(w350) -> ("State"=w360:T9)
            n129 = case shown="\"Measuring\", Default" w360 {
              tunnel: [w367 w373] -> w356
              tunnel: w351 -> [w363 w373]
              tunnel: w362 -> [_ _]
              tunnel: w361 -> [w371 _]
              tunnel: w350 -> [w365 w372]
              tunnel: [w369 w372] -> w349
              frame "Measuring", Default {
                # "If the system is logging, stop logging."
                n130 = call "Close.vi"("error in (no error)"=w363, "State in"=w365) -> ("error out"=w364:errorcluster, "State out"=w366:T13)  [unwired: 8 in]
                n131 = Bundle By Name(cluster=w366, "State"=State_Enum."Idle") -> (w369:T13)
                n132 = call-poly "Enqueue Message.vi"("error in (no error)"=w364, "Message"="Logging Stopped", "Message Queue"=w371) -> ("error out"=w367:errorcluster)  [unwired: 7 in, 1 out]
              }
              frame "Idle" {
                # "The system is already idle. Ignore the \"Stop\" message."
              }
            }
            n133 = call-poly "Enqueue Message.vi"("error in (no error)"=w356, "Message Data"=w349, "Message"="Update", "Message Queue"=w353) -> ("error out"=w357:errorcluster)  [unwired: 6 in, 1 out]
            n134 = call-poly "Enqueue Message.vi"("error in (no error)"=w357, "Message Data"=w352, "Message"="Update", "Message Queue"=w354) -> ("error out"=w355:errorcluster)  [unwired: 6 in, 1 out]
          }
          frame "Pause" {
            # "Stop - Flush the message queue of any pending \"Log\" messages. Call 'Flush Data to Log File.vi' so any pending data is not lost."
            n135 = Unbundle By Name(w379) -> ("State"=w385:T9, "First Iteration"=w378:bool)
            n136 = case shown="True" w378 {
              tunnel: w379 -> [w388 w393]
              tunnel: [w388 w394] -> w375
              tunnel: w377 -> [w387 w391]
              tunnel: [w387 w390] -> w376
              frame False {
              }
              frame True {
                # "If we load to a paused state we initialize"
                n137 = call "Initialize.vi"("error in (no error)"=w391, "State in"=w393) -> ("error out"=w390:errorcluster, "Pump Initialized"=w395:bool, "State out"=w392:T13)  [unwired: 7 in]
                n138 = case shown="False" w395 {
                  tunnel: [enum16{"Off", "On", "Not Initialized"}."Not Initialized" ("Pump On?") enum16{"Off", "On", "Not Initialized"}."Off" ("Pump On?")] -> w396
                  tunnel: [TRUE FALSE] -> w389
                  frame False {
                  }
                  frame True {
                  }
                }
                n139 = Bundle By Name(cluster=w392, "Pump On?"=w396, "First Iteration"=w389) -> (w394:T13)
              }
            }
            n140 = case shown="\"Measuring\", Default" w385 {
              tunnel: [w405 w413 w417] -> w382
              tunnel: w376 -> [w403 w413 w417]
              tunnel: w386 -> [w409 _ _]
              tunnel: w375 -> [w404 w411 w415]
              tunnel: [w407 w410 w414] -> w374
              frame "Measuring", Default {
                # "If the system is logging, stop logging."
                n141 = call "Pause.vi"("error in (no error)"=w403, "State in"=w404) -> ("error out"=w402:errorcluster, "State out"=w401:T13)  [unwired: 8 in]
                n142 = Bundle By Name(cluster=w401, "State"=State_Enum."Paused") -> (w407:T13)
                n143 = call-poly "Enqueue Message.vi"("error in (no error)"=w402, "Message"="Logging Stopped", "Message Queue"=w409) -> ("error out"=w405:errorcluster)  [unwired: 7 in, 1 out]
              }
              frame "Idle" {
                # "The system is already idle. Ignore the \"Stop\" message."
                n144 = Bundle By Name(cluster=w411, "State"=State_Enum."Paused") -> (w410:T13)
              }
              frame "Paused" {
                n145 = Bundle By Name(cluster=w415, "State"=State_Enum."Paused") -> (w414:T13)
              }
            }
            n146 = call-poly "Enqueue Message.vi"("error in (no error)"=w382, "Message Data"=w380, "Message"="Update", "Message Queue"=w383) -> ("error out"=w381:errorcluster)  [unwired: 6 in, 1 out]
          }
          frame "Update Settings" {
            # "New settings are available, update the current ones stored in the shift register with the settings sent as part of the message"
            n147 = Variant To Data(error in=w424, type=T10 {"Cycle Period"=500.0, "PID 2 Parameters"={"Input Device"=enum."Default", "Output Device"=enum."Equilibar Pressure Reg", "Setpoint"=0.0, "PID gains"={"proportional gain (Kc)"=1.0, "integral time (Ti, min)"=0.01, "derivative time (Td, min)"=0.0}, "output range"={"output low"=0.0, "output high"=100.0}}, "Manual Entry"=0.0, "Auto?"=TRUE, "4-20mA Input Settings"={"Input Channel "=0}, "4-20mA Out Settings"={"Output DAQ Task"=""}, "Input Channel Tag Name "=""} ("Settings"), Variant=w425) -> (data=w419:T10, error out=w422:errorcluster)
            n148 = Bundle By Name(cluster=w421, "Configuration"=w419) -> (w418:T13)
          }
          frame "Exit" {
            # "Release the Logging queue reference"
            # "Don't check the error out. The UI message queue may have already been released."
            # "Stop the VI"
            # "Exit - Send the Exit message to the UI Message Handler.  Call 'Flush Data to Log File.vi' so any pending data is not lost."
            n149 = Release Queue(queue=w430, error in (no error)=w433) -> (error out=w429:errorcluster)  [unwired: 1 in, 2 out]
            n150 = call-poly "Enqueue Message.vi"("Priority Message? (F)"=TRUE, "Message"="Exit", "Message Queue"=w434) -> ("error out"=w428:errorcluster)  [unwired: 7 in, 1 out]
            n151 = call <vilib>:"Clear Errors.vi"("error in (no error)"=w428) -> ()  [unwired: 5 in, 2 out]
            n152 = Merge Errors(w429) -> (w435:errorcluster)
          }
          frame "---Copy This Frame---" {
            # "Duplicate this frame when creating new messages.  Change this comment in the duplicated frame to describe this message."
            n153 = Merge Errors(w440) -> (w439:errorcluster)
          }
          frame Default {
            # "'Default' case only runs if there is a message that isn't defined in any of the other cases.  Output a programming error."
            n154 = xnode "Error Ring"("parameter 0"=w443) -> ("error out"=w444:errorcluster)
          }
        }
        n155 = Unbundle By Name(w17) -> ("State"=w31:T9, "Configuration.Cycle Period"=w29:dbl)
        n156 = call "Error Handler.vi"("error in (no error)"=w37, "Message Queue"=w35) -> ("dup error in"=w36:errorcluster)  [unwired: 8 in, 1 out]
        n157 = case shown="\"Paused\"" w31 {
          tunnel: [w43 1 1] -> w30
          tunnel: w29 -> [w43 _ _]
          frame "Measuring" {
          }
          frame "Idle" {
          }
          frame "Paused" {
          }
        }
        n158 = node-c288(w30) -> ()  [unwired: 1 in, 1 out]
      }
      n159 = node-c288(w12) -> ()  [unwired: 1 out]
    }
    frame Error {
    }
  }
  "error out" <- w3
